vi "select spot to track.vi"(10 "new circle":bool, 11 "N spot tracker in":T1) -> (1 "use photons to track":bool, 2 "state transition":bool, 3 "N spot tracker out":T1)   [LabVIEW 2010]
uses:
  kalman N spot state.ctl
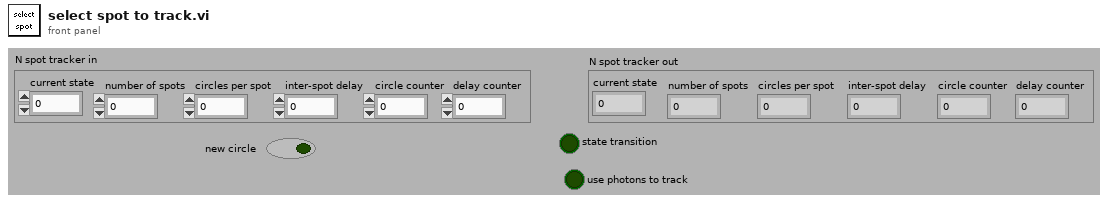
[diagram p1: front panel]
types:
  T1 = typedef "kalman N spot state.ctl" = cluster{"current state":u8, "number of spots":u8, "circles per spot":u16, "inter-spot delay":u8, "circle counter":u16, "delay counter":u8}
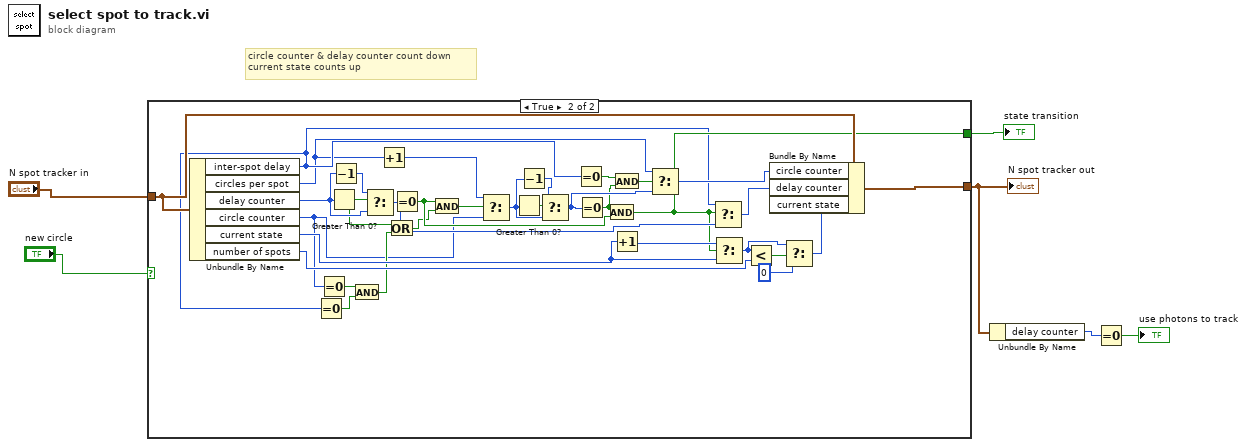
[diagram p0: block diagram]
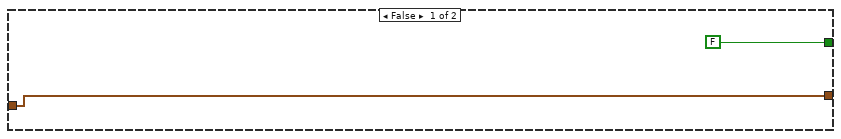
[diagram p2: hidden frame]
diagram:
  # "circle counter & delay counter count down\ncurrent state counts up"
  n1 = case shown="True" "new circle" {
    tunnel: "N spot tracker in" -> [w7 w26]
    tunnel: [w7 w27] -> w1
    tunnel: [FALSE w24] -> w5
    frame False {
    }
    frame True {
      n2 = Unbundle By Name(w26) -> ("inter-spot delay"=w13:u8, "circles per spot"=w12:u16, "delay counter"=w25:u8, "circle counter"=w16:u16, "current state"=w34:u8, "number of spots"=w33:u8)
      n3 = Equal To 0?(x=w13) -> (x = 0?=w19:bool)
      n4 = Equal To 0?(x=w16) -> (x = 0?=w20:bool)
      n5 = Greater Than 0?(x=w25) -> (x > 0?=w21:bool)
      n6 = Decrement(x=w25) -> (x-1=w41:u8)
      n7 = And(x=w20, y=w19) -> (x .and. y?=w17:bool)
      n8 = Select(t=w41, s=w21, f=w25) -> (s? t:f=w36:u8)
      n9 = Increment(x=w12) -> (x+1=w22:u16)
      n10 = Or(x=w21, y=w17) -> (x .or. y?=w18:bool)
      n11 = Equal To 0?(x=w36) -> (x = 0?=w23:bool)
      n12 = And(x=w23, y=w18) -> (x .and. y?=w40:bool)
      n13 = Select(t=w22, s=w40, f=w16) -> (s? t:f=w38:u16)
      n14 = Greater Than 0?(x=w38) -> (x > 0?=w37:bool)
      n15 = Decrement(x=w38) -> (x-1=w39:u16)
      n16 = Select(t=w39, s=w37, f=w38) -> (s? t:f=w14:u16)
      n17 = Equal To 0?(x=w13) -> (x = 0?=w10:bool)
      n18 = Equal To 0?(x=w14) -> (x = 0?=w9:bool)
      n19 = And(x=w9, y=w23) -> (x .and. y?=w24:bool)
      n20 = And(x=w10, y=w9) -> (x .and. y?=w11:bool)
      n21 = Increment(x=w34) -> (x+1=w35:u8)
      n22 = Select(t=w12, s=w11, f=w14) -> (s? t:f=w15:u16)
      n23 = Select(t=w13, s=w24, f=w36) -> (s? t:f=w28:u8)
      n24 = Select(t=w35, s=w24, f=w34) -> (s? t:f=w31:u8)
      n25 = Less?(x=w31, y=w33) -> (x < y?=w32:bool)
      n26 = Select(t=w31, s=w32, f=u8 0) -> (s? t:f=w29:u8)
      n27 = Bundle By Name(cluster=w26, "circle counter"=w15, "delay counter"=w28, "current state"=w29) -> (w27:T1)
    }
  }
  "state transition" <- w5
  "N spot tracker out" <- w1
  n28 = Unbundle By Name(w1) -> ("delay counter"=w2:u8)
  n29 = Equal To 0?(x=w2) -> (x = 0?=→"use photons to track":bool)
